vi "Fit.vi"(8 "error in (no error)":errorcluster caption="entrée d'erreur (pas d'erreur)", 9 "y":string[][](array[string]), 10 "X":string[][](array[string]), 11 "RobustScaler.lvclass":refnum<class "RobustScaler.lvclass">) -> (0 "error out":errorcluster caption="sortie d'erreur", 2 "String Data":string, 3 "RobustScaler.lvclass":refnum<class "RobustScaler.lvclass">)   [LabVIEW 2020, in "RobustScaler.lvclass"]
doc: "Compute the median and quantiles to be used for scaling.\n\nReturns : \n\n- String : OK"
uses:
  RobustScaler.lvclass
  RobustScaler.lvclass/RobustScaler.ctl
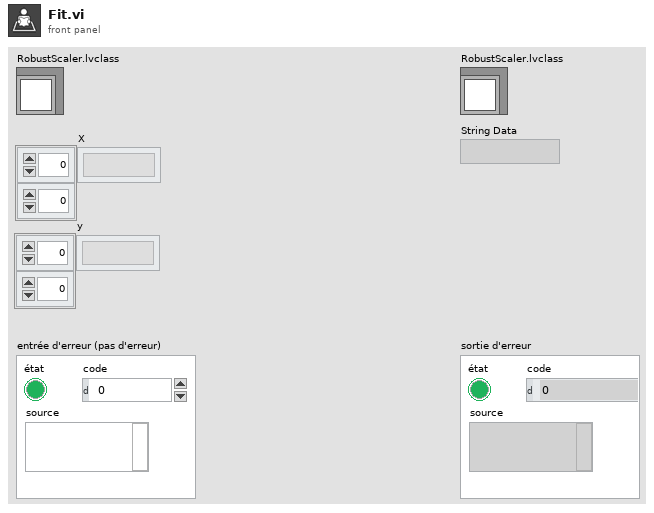
[diagram p1: front panel]
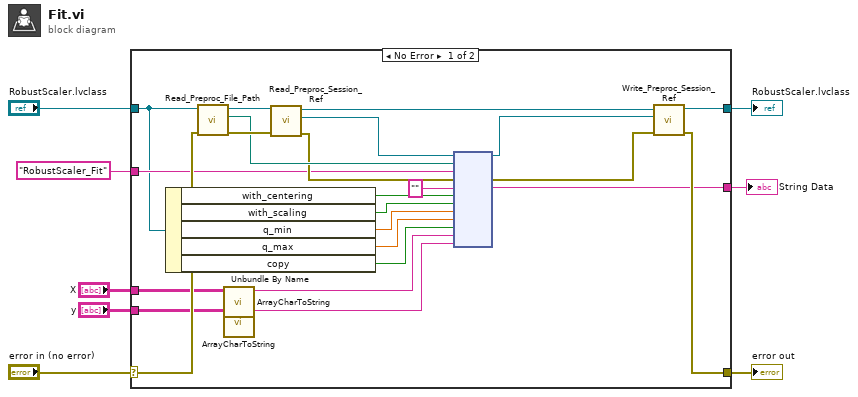
[diagram p0: block diagram]
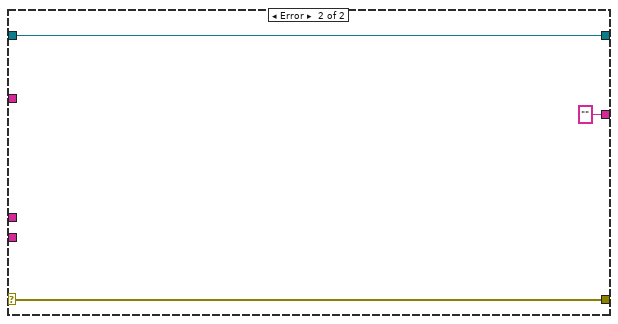
[diagram p2: hidden frame]
diagram:
  n1 = case shown="No Error" "error in (no error)" {
    selector: "error in (no error)" -> [w18 w35]
    tunnel: [w19 w35] -> w7
    tunnel: [w20 w34] -> w5
    tunnel: "RobustScaler.lvclass" -> [w15 w34]
    tunnel: "RobustScaler_Fit" ("Fonction") -> [w17 _]
    tunnel: [w16 ""] -> w3
    tunnel: "X" -> [w12 _]
    tunnel: "y" -> [w10 _]
    frame No Error {
      n2 = Unbundle By Name(w15) -> ("with_centering"=w23:bool, "with_scaling"=w22:bool, "q_min"=w21:dbl, "q_max"=w14:dbl, "copy"=w13:bool)
      n3 = call-dynamic "Read_Preproc_File_Path.vi"("error in (no error)"=w18, "Python in"=w15) -> ("error out"=w31:errorcluster, "File_Path"=w28:path, "Python out"=w32:refnum<class "RobustScaler.lvclass">)  [unwired: 7 in]
      n4 = call "ArrayCharToString.vi"("TAB"=w12) -> ("Instruction"=w11:string)  [unwired: 10 in]
      n5 = call "ArrayCharToString.vi"("TAB"=w10) -> ("Instruction"=w9:string)  [unwired: 10 in]
      n6 = call-dynamic "Read_Preproc_Session_Ref.vi"("error in (no error)"=w31, "Python in"=w32) -> ("error out"=w27:errorcluster, "Session_ref"=w29:refnum<k35>, "Python out"=w30:refnum<class "RobustScaler.lvclass">)  [unwired: 7 in]
      n7 = node(w29, w28, w17, w27, "", w23, w22, w21, w14, w13, w11, w9) -> (w25:refnum<k35>, w26:errorcluster, w16:string)  [unwired: 7 in, 2 out]
      n8 = call-dynamic "Write_Preproc_Session_Ref.vi"("error in (no error)"=w26, "Session_ref"=w25, "Python in"=w30) -> ("error out"=w19:errorcluster, "Python out"=w20:refnum<class "RobustScaler.lvclass">)  [unwired: 7 in]
    }
    frame Error {
    }
  }
  "error out" <- w7
  "RobustScaler.lvclass" <- w5
  "String Data" <- w3
